vi "Ciclo for Bool.vi"() -> ()   [LabVIEW 2012]
panel:
  out "Array 2":dbl[](array[numeric])
  out "Numeric":dbl format="%#_1g"
  out "Boolean":bool
  out "Array":bool[](array[boolean])
  # "Realizzare un VI che utilizza un ciclo FOR che genera 5 numeri casuali\ne accende il LED se il numero generato  >0.5.\nVisualizzare istantaneamente inisieme il booleano, il valeore del numero\ngenerato e dell'iterazione"
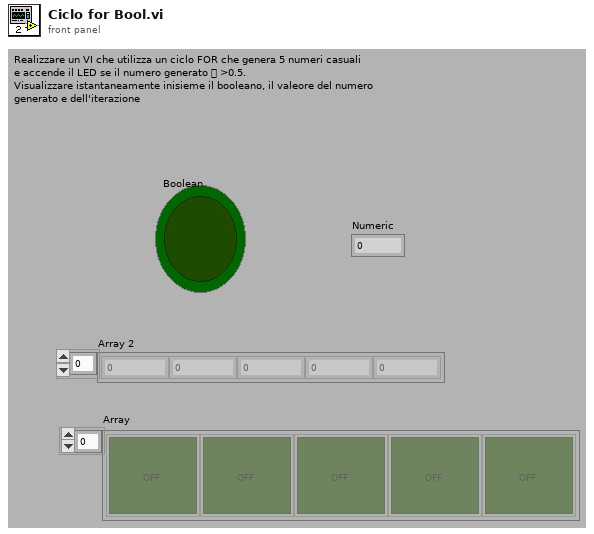
[diagram p1: front panel]
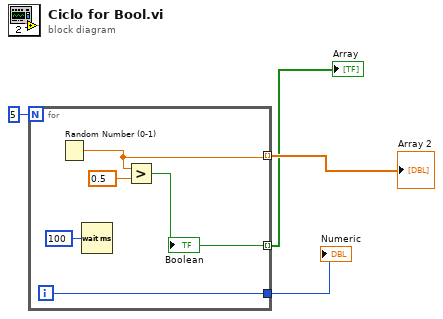
[diagram p0: block diagram]
diagram:
  n1 = for {
    N: 5 -> [_]
    tunnel: [w8] -> w3
    tunnel: [w6] -> w2 mode=indexing
    tunnel: [w5] -> w1 mode=indexing
    i -> [w8]
    n2 = Random Number (0-1)() -> (number: 0 to 1=w6:dbl)
    n3 = Wait (ms)(milliseconds to wait=100) -> ()  [unwired: 1 out]
    n4 = Greater?(x=w6, y=0.5) -> (0:w5:bool)
    "Boolean" <- w5
  }
  "Array" <- w1
  "Numeric" <- w3
  "Array 2" <- w2
